vi "Display Error.vi"(2 "Error Type":enum16{"Channel Error", "Label Error"}(ring)=enum."Label Error", 7 "Errors":string[](array[string])) -> ()   [LabVIEW 2017]
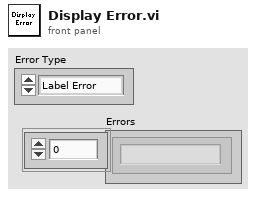
[diagram p1: front panel]
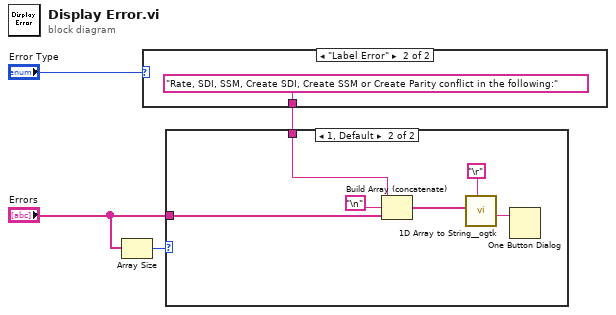
[diagram p0: block diagram]
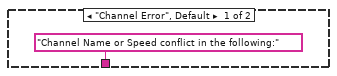
[diagram p2: hidden frame]
diagram:
  n1 = Array Size(array="Errors") -> (size(s)=w3:i32)
  n2 = case shown="\"Label Error\"" "Error Type" {
    tunnel: ["Channel Name or Speed conflict in the following:" ("string") "Rate, SDI, SSM, Create SDI, Create SSM or Create Parity conflict in the following:" ("string")] -> w1
    frame "Channel Error", Default {
    }
    frame "Label Error" {
    }
  }
  n3 = case shown="1, Default" w3 {
    tunnel: "Errors" -> [_ w8]
    tunnel: w1 -> [_ w7]
    frame 0 {
    }
    frame 1, Default {
      n4 = Build Array (concatenate)(w7, "\n", w8) -> (w10:string[])
      n5 = call <userlib>:"1D Array to String__ogtk.vi"("delimiter (Tab)"="\r", "Array of Strings"=w10) -> ("delimited string"=w11:string)  [unwired: 9 in]
      n6 = One Button Dialog(message=w11) -> ()  [unwired: 1 in, 1 out]
    }
  }
